vi "GetAttribute1.vi"(0 "reference in":refnum<class "G#SubClass1.lvclass">, 5 "error in (no error)":errorcluster) -> (14 "reference out":refnum<class "G#SubClass1.lvclass">, 15 "Base class.Numeric":dbl, 16 "SubAttribute":dbl, 17 "Base class.Array":dbl[](array[numeric]), 19 "error out":errorcluster)   [LabVIEW 2017, in "G#SubClass1.lvclass"]
uses:
  G#SubClass1.lvclass
  C:/Projects/GsharpGIT2017/Verification/TestCases/TestClasses/G#BaseClass1_class/G#BaseClass1.lvclass
  G#BaseClass1_class/G#BaseClass1.lvclass
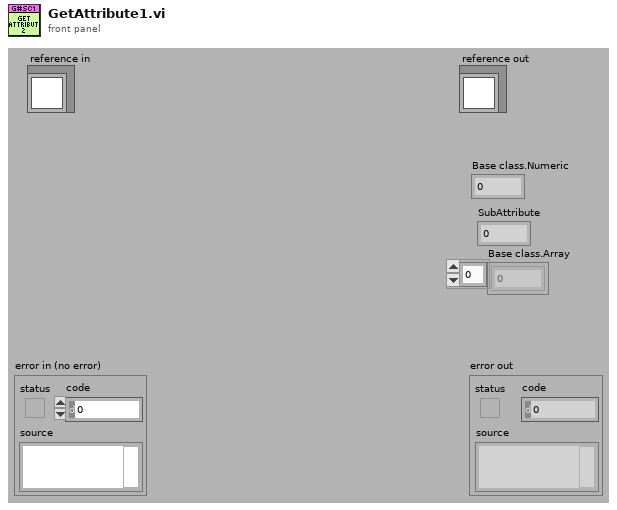
[diagram p1: front panel]
types:
  T1 = typedef "G#SubClass1.lvclass/ObjectAttributes.ctl" = cluster{"SubNumeric":dbl, "TestQueue":refnum<queue>}
  T2 = typedef "G#BaseClass1.lvclass/ObjectAttributes.ctl" = cluster{"Numeric":dbl, "Array":dbl[]}
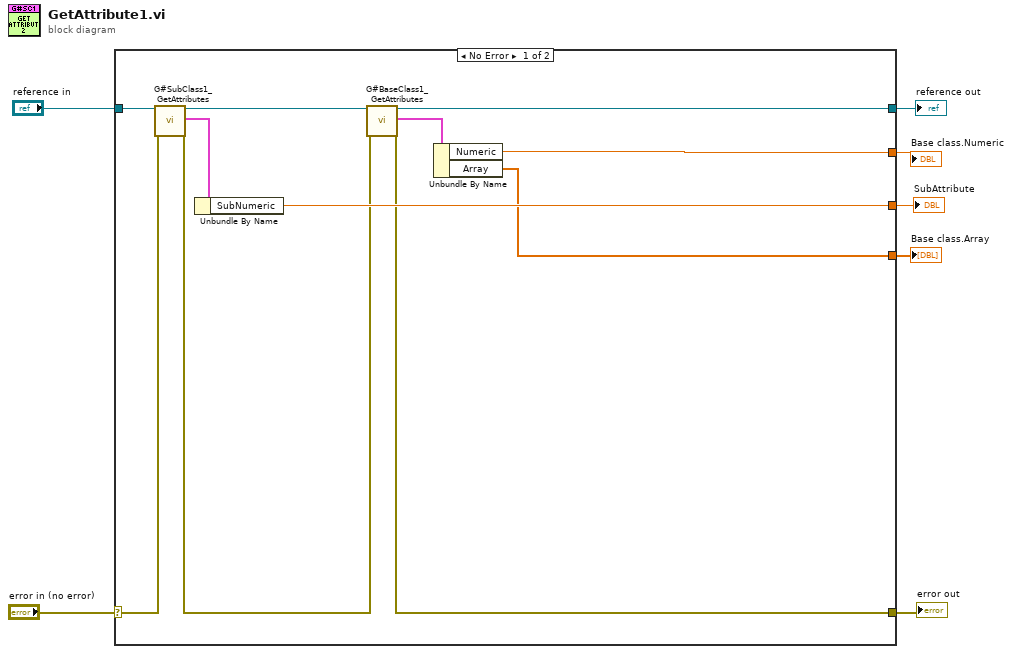
[diagram p0: block diagram]
diagram:
  n1 = case shown="No Error" "error in (no error)" {
    selector: "error in (no error)" -> [w18 w20]
    tunnel: [w11 w20] -> w6
    tunnel: [w13 w19] -> w4
    tunnel: "reference in" -> [w16 w19]
    tunnel: [w15 _] -> w3
    tunnel: [w9 _] -> w2
    tunnel: [w8 _] -> w1
    frame No Error {
      n2 = call "G#SubClass1_GetAttributes.vi"("reference in"=w16, "error in (no error)"=w18) -> ("reference out"=w14:refnum<class "G#SubClass1.lvclass">, "attributes"=w17:T1, "error out"=w12:errorcluster)  [unwired: 14 in, 1 out]
      n3 = Unbundle By Name(w17) -> ("SubNumeric"=w15:dbl)
      n4 = call "G#BaseClass1_GetAttributes.vi"("reference in"=w14, "error in (no error)"=w12) -> ("reference out"=w13:refnum<class "G#SubClass1.lvclass">, "attributes"=w10:T2, "error out"=w11:errorcluster)  [unwired: 14 in, 1 out]
      n5 = Unbundle By Name(w10) -> ("Numeric"=w9:dbl, "Array"=w8:dbl[])
    }
    frame Error {
    }
  }
  "error out" <- w6
  "reference out" <- w4
  "Base class.Numeric" <- w2
  "SubAttribute" <- w3
  "Base class.Array" <- w1
